vi "ZCR_enhanced_measurement_v6.vi"(8 "error in (no error)":errorcluster, 9 "Relay":enum16{"R1", "R2"}(ring), 10 "Serial Number":string, 11 "ZCR Signal Input":waveform(dbl)[](graph)=[{"t0"=timestamp(3707890383.8976955 s since 1904-01-01), "dt"=9.999999999999999e-05, "Y"=array[20000 elements], "attributes"=variant("NI_ChannelName"=variant(string "Tension_0"), "NI_UnitDescription"=variant(string "Volts"))}, {"t0"=timestamp(3707890383.8977456 s since 1904-01-01), "dt"=9.999999999999999e-05, "Y"=array[20000 elements], "attributes"=variant("NI_ChannelName"=variant(string "Tension_1"), "NI_UnitDescription"=variant(string "Volts"))}] caption="ZCR signal imput") -> (0 "error out":errorcluster, 1 "SIN OFF (x10)ms":dbl format="%0.2f", 2 "SIN ON (x10)ms":dbl format="%0.2f", 3 "ZCR measure OK ?":bool, 4 "Reglage decalage":T1={"Delta relais On (Secondes)"=0.002411111111111111, "Delta relais  Off(Secondes)"=0.0007555555555555556})   [LabVIEW 2020, in "Library Commun.lvlib" / "Nodon_ZCR.lvclass"]
uses:
  Nodon_ZCR.lvclass
  <vilib>/Utility/miscctls.llb/LVRangeTypeDef.ctl
  <vilib>/Analysis/baseanly.llb/Mean (DBL).vi
  <vilib>/Analysis/NI_AALBase.lvlib
  Library Commun.lvlib
panel:
  out "SIN ON Points":i32[](array[numeric])
  out "SIN OFF Points":i32[](array[numeric])
  out "ZCR OFF":waveform(dbl)[](graph)=[{"t0"=timestamp(3707890383.8976955 s since 1904-01-01), "dt"=9.999999999999999e-05, "Y"=array[20000 elements], "attributes"=variant("NI_ChannelName"=variant(string "Tension_0"), "NI_UnitDescription"=variant(string "Volts"))}, {"t0"=timestamp(3707890383.8977456 s since 1904-01-01), "dt"=9.999999999999999e-05, "Y"=array[20000 elements], "attributes"=variant("NI_ChannelName"=variant(string "Tension_1"), "NI_UnitDescription"=variant(string "Volts"))}]
  out "Input Signal":waveform(dbl)[](graph)=[{"t0"=timestamp(3810040522.776 s since 1904-01-01), "dt"=0.0002, "Y"=array[5000 elements]}, {"t0"=timestamp(3810040522.777 s since 1904-01-01), "dt"=0.0002, "Y"=array[5000 elements]}]
  out "SIN OFF Delay":i32[](array[numeric])
  out "SIN ON Delay":i32[](array[numeric])
  # "ZCR Enhanced V5"
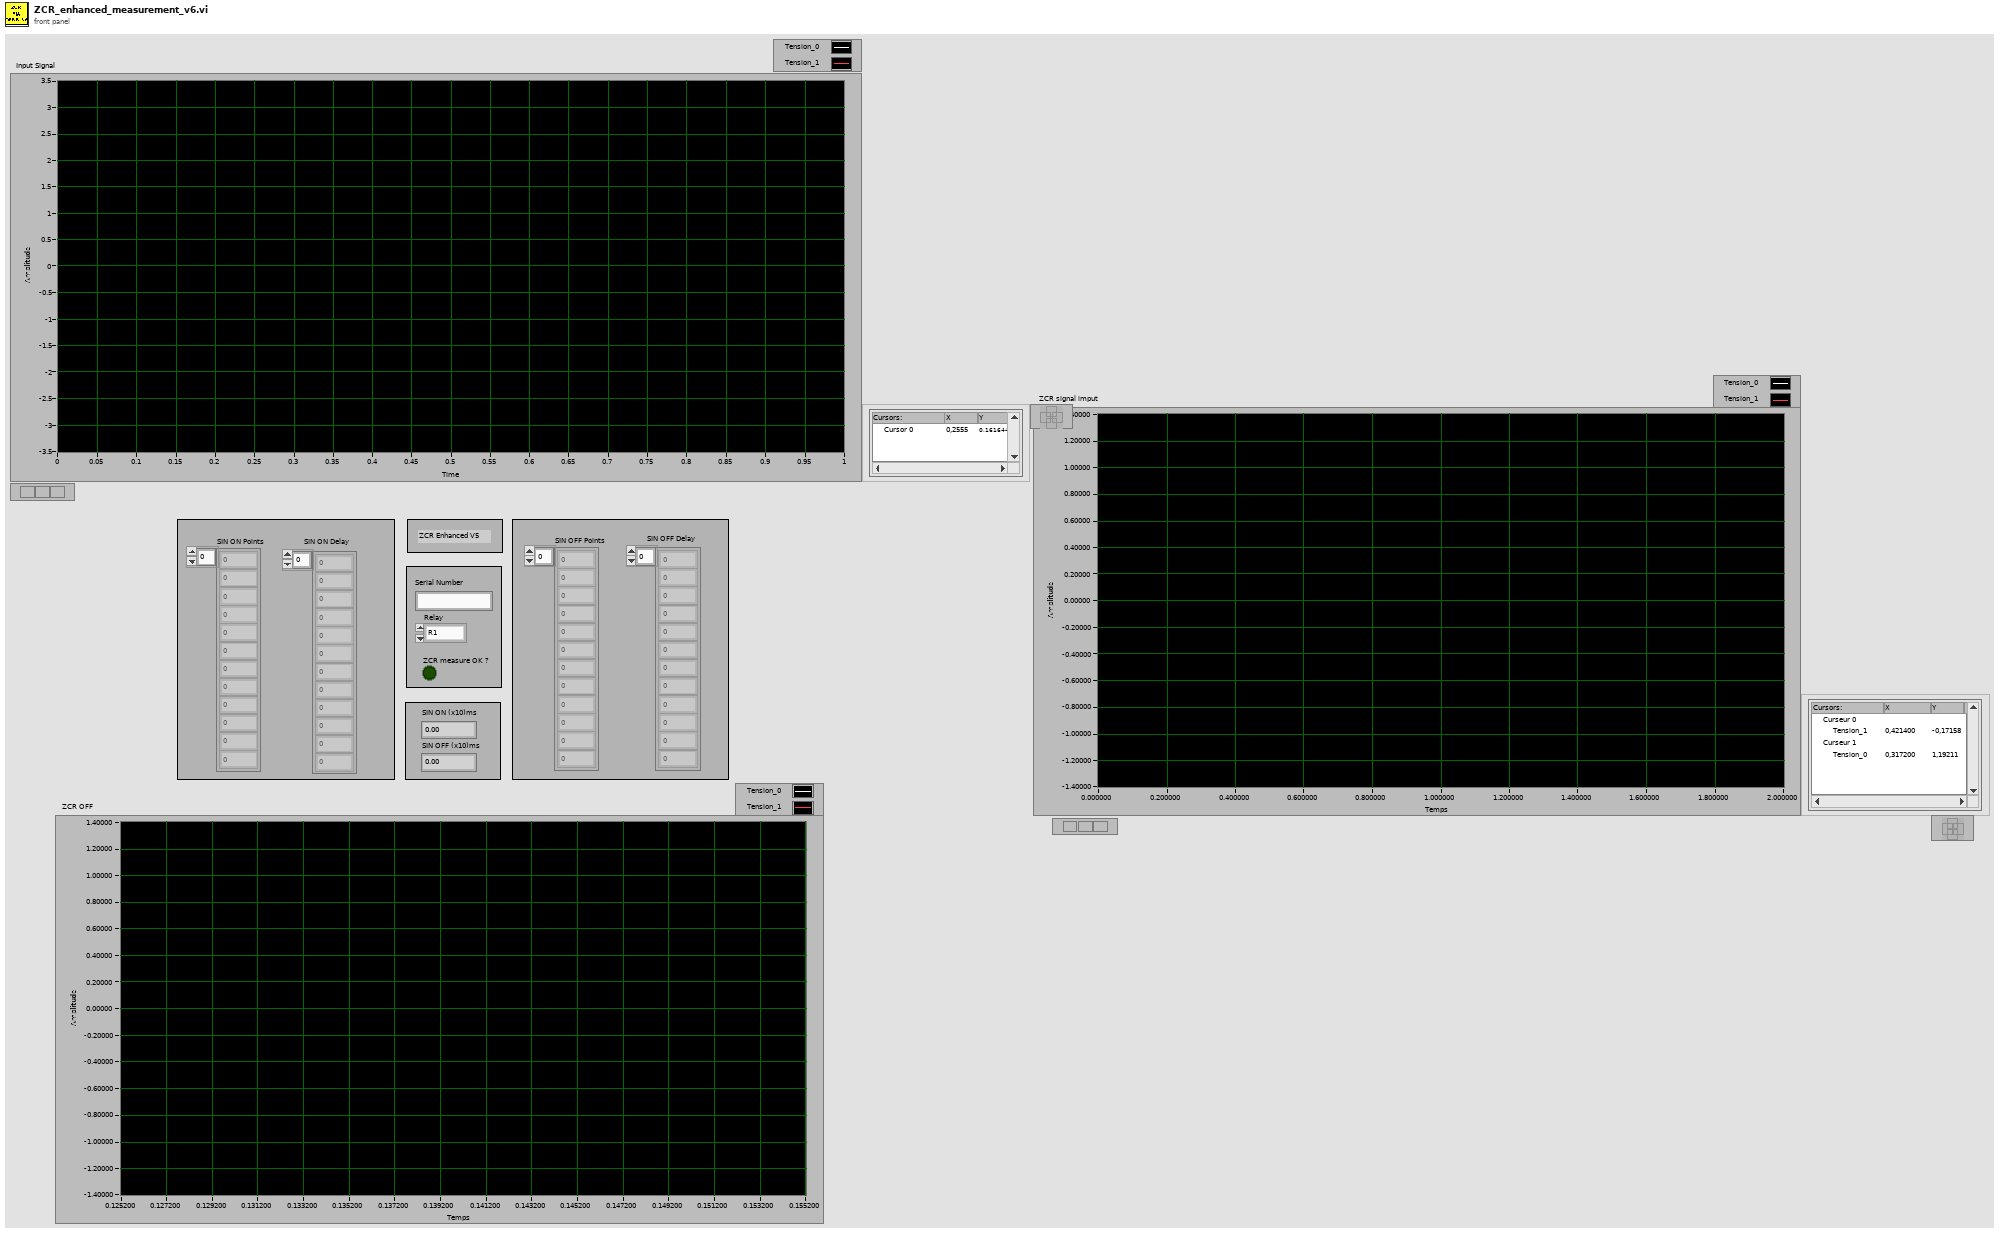
[diagram p1: front panel]
types:
  T1 = cluster{"Delta relais On (Secondes)":dbl, "Delta relais  Off(Secondes)":dbl}
  T2 = typedef "LVRangeTypeDef.ctl" = cluster{"Minimum":dbl, "Maximum":dbl, "Increment":dbl, "Minor Increment":dbl, "Start":dbl}
  T3 = typedef "imagedata.ctl" = cluster{"image type":i32, "image depth":i32, "image":u8[], "mask":u8[], "colors":u32[], "Rectangle":cluster{"left":i16, "top":i16, "right":i16, "bottom":i16}}
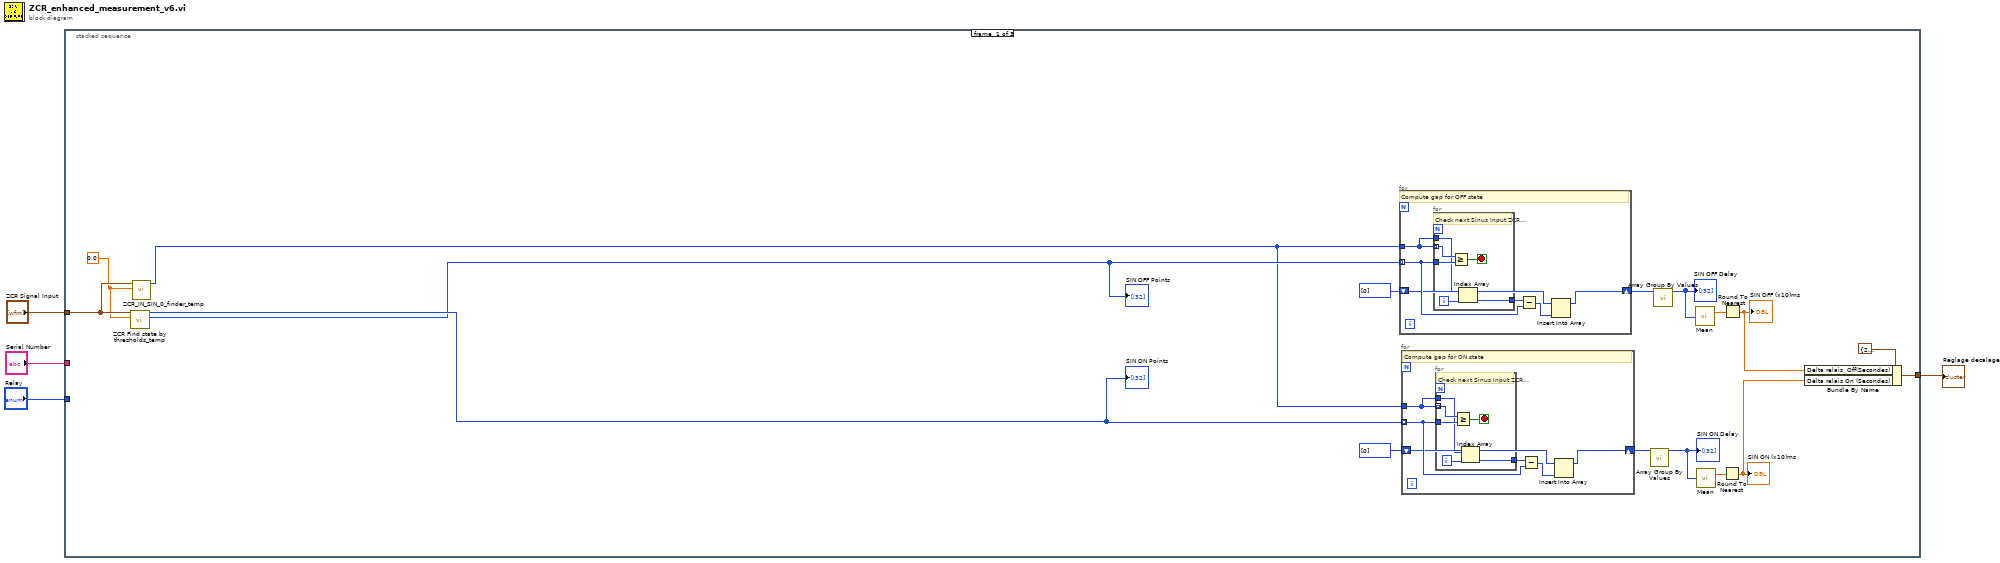
[diagram p0: block diagram]
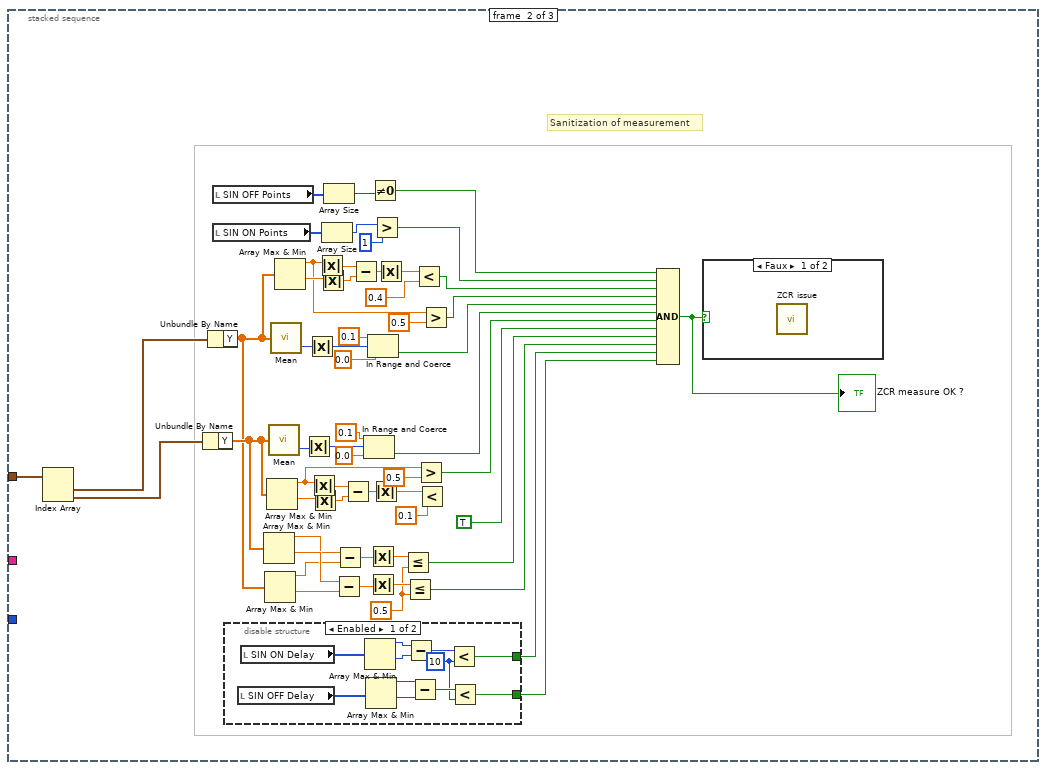
[diagram p2: hidden frame]
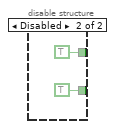
[diagram p3: hidden frame]
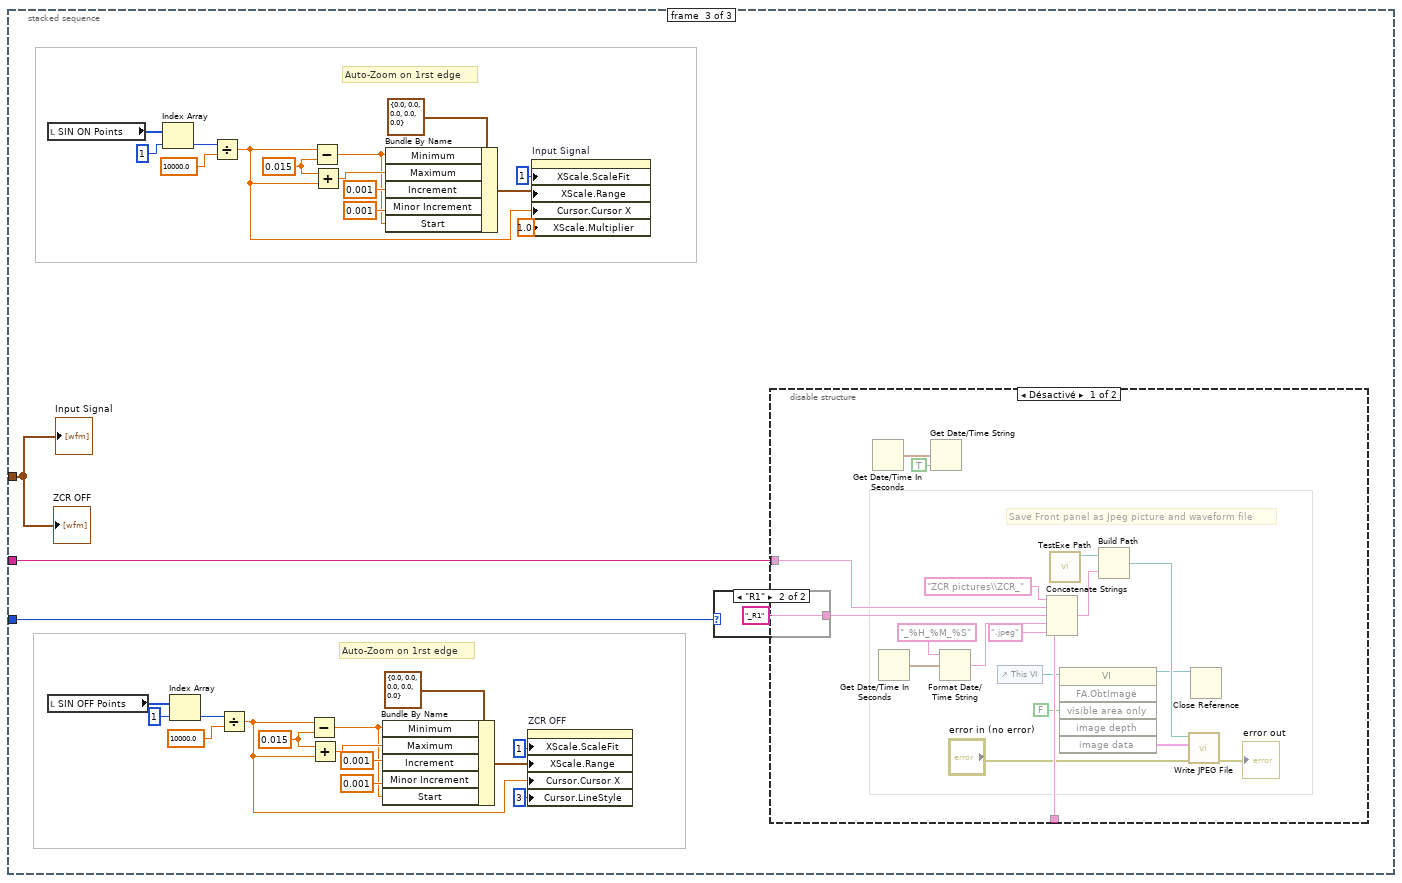
[diagram p5: hidden frame]
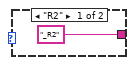
[diagram p7: hidden frame]
diagram:
  n1 = stacked-sequence {
    tunnel: "ZCR Signal Input" -> [w10 w47 w115]
    tunnel: "Serial Number" -> [_ _ w116]
    tunnel: "Relay" -> [_ _ w118]
    tunnel: [w15 _ _] -> w1
    frame #0 {
      w8 = 0.0
      n2 = call "ZCR Find state by thresholds_temp.vi"("Noise amplitude"=w8, "Input Signal"=w10) -> ("SIN OFF Points"=w11:i32[], "SIN ON Points"=w12:i32[])  [unwired: 8 in]
      "SIN OFF Points" <- w11
      "SIN ON Points" <- w12
      n3 = call "ZCR_IN_SIN_0_finder_temp.vi"("Noise amplitude"=w8, "ZCR IN"=w10) -> ("OFF SIN"=w9:i32[])  [unwired: 9 in]
      n4 = for {
        tunnel: w11 -> [w25] mode=indexing
        tunnel: w9 -> [w27]
        shift-right: [w22] -> w6
        shift-left: i32[] [0] -> [w24]
        # "Compute gap for OFF state"
        n5 = for {
          tunnel: w27 -> [w33] mode=indexing
          tunnel: w25 -> [w32]
          tunnel: w27 -> [w30]
          tunnel: [w29] -> w26
          i -> [w28]
          stop <- w31 stop-if-true
          # "Check next Sinus Input ZCR crossing"
          n6 = Greater Or Equal?(x=w33, y=w32) -> (x >= y?=w31:bool)
          n7 = Index Array(array=w30, index=w28) -> (element=w29:i32)
        }
        n8 = Subtract(x=w26, y=w25) -> (x-y=w23:i32)
        n9 = Insert Into Array(array=w24, new element=w23) -> (w22:i32[])  [unwired: 1 in]
      }
      n10 = for {
        tunnel: w12 -> [w37] mode=indexing
        tunnel: w9 -> [w39]
        shift-right: [w34] -> w19
        shift-left: i32[] [0] -> [w36]
        # "Compute gap for ON state"
        n11 = for {
          tunnel: w39 -> [w45] mode=indexing
          tunnel: w37 -> [w44]
          tunnel: w39 -> [w42]
          tunnel: [w41] -> w38
          i -> [w40]
          stop <- w43 stop-if-true
          # "Check next Sinus Input ZCR crossing"
          n12 = Greater Or Equal?(x=w45, y=w44) -> (x >= y?=w43:bool)
          n13 = Index Array(array=w42, index=w40) -> (element=w41:i32)
        }
        n14 = Subtract(x=w38, y=w37) -> (x-y=w35:i32)
        n15 = Insert Into Array(array=w36, new element=w35) -> (w34:i32[])  [unwired: 1 in]
      }
      n16 = call "Array Group By Values.vi"("Input Array"=w19) -> ("Output Value"=w7:i32[])  [unwired: 10 in]
      "SIN ON Delay" <- w7
      n17 = call "Array Group By Values.vi"("Input Array"=w6) -> ("Output Value"=w5:i32[])  [unwired: 10 in]
      "SIN OFF Delay" <- w5
      n18 = call-poly <vilib>:"Mean.vi"("X"=w5) -> ("mean"=w17:dbl)  [unwired: 1 out]
      n19 = call-poly <vilib>:"Mean.vi"("X"=w7) -> ("mean"=w18:dbl)  [unwired: 1 out]
      n20 = Round To Nearest(number=w18) -> (nearest integer value=w13:dbl)
      "SIN ON (x10)ms" <- w13
      n21 = Round To Nearest(number=w17) -> (nearest integer value=w14:dbl)
      "SIN OFF (x10)ms" <- w14
      n22 = Bundle By Name(cluster=T1 {"Delta relais On (Secondes)"=24.0, "Delta relais  Off(Secondes)"=7.0} ("Reglage decalage"), "Delta relais  Off(Secondes)"=w14, "Delta relais On (Secondes)"=w13) -> (w15:T1)
    }
    frame #1 {
      w55 = 0.5
      # "Sanitization of measurement"
      n23 = Index Array(array=w47) -> (element #1=w98:waveform(dbl), element #2=w97:waveform(dbl))  [unwired: 2 in]
      n24 = Unbundle By Name(w97) -> ("Y"=w65:dbl[])
      n25 = Unbundle By Name(w98) -> ("Y"=w64:dbl[])
      n26 = local read "SIN OFF Points"() -> (w101:i32[])
      n27 = local read "SIN ON Points"() -> (w100:i32[])
      n28 = disable-structure shown="Enabled" {
        disable-tunnel: [w103 TRUE] -> w49
        disable-tunnel: [w102 TRUE] -> w48
        frame Enabled {
          w104 = 10 ("y")
          n29 = local read "SIN OFF Delay"() -> (w111:i32[])
          n30 = local read "SIN ON Delay"() -> (w112:i32[])
          n31 = Array Max & Min(array=w112) -> (max value=w109:i32, min value=w110:i32)  [unwired: 2 out]
          n32 = Array Max & Min(array=w111) -> (max value=w107:i32, min value=w108:i32)  [unwired: 2 out]
          n33 = Subtract(x=w109, y=w110) -> (x-y=w106:i32)
          n34 = Subtract(x=w107, y=w108) -> (x-y=w105:i32)
          n35 = Less?(x=w106, y=w104) -> (x < y?=w103:bool)
          n36 = Less?(x=w105, y=w104) -> (x < y?=w102:bool)
        }
        frame Disabled {
        }
      }
      n37 = Array Max & Min(array=w65) -> (max value=w61:dbl, min value=w63:dbl)  [unwired: 2 out]
      n38 = Array Max & Min(array=w64) -> (max value=w60:dbl, min value=w62:dbl)  [unwired: 2 out]
      n39 = Array Max & Min(array=w65) -> (max value=w78:dbl, min value=w88:dbl)  [unwired: 2 out]
      n40 = call-poly <vilib>:"Mean.vi"("X"=w65) -> ("error"=w95:i32)  [unwired: 1 out]
      n41 = call-poly <vilib>:"Mean.vi"("X"=w64) -> ("error"=w96:i32)  [unwired: 1 out]
      n42 = Array Max & Min(array=w64) -> (max value=w75:dbl, min value=w83:dbl)  [unwired: 2 out]
      n43 = Absolute Value(x=w95) -> (abs(x)=w93:i32)
      n44 = Absolute Value(x=w96) -> (abs(x)=w94:i32)
      n45 = Absolute Value(x=w78) -> (abs(x)=w86:dbl)
      n46 = Absolute Value(x=w88) -> (abs(x)=w87:dbl)
      n47 = Absolute Value(x=w75) -> (abs(x)=w81:dbl)
      n48 = Absolute Value(x=w83) -> (abs(x)=w82:dbl)
      n49 = Array Size(array=w100) -> (size(s)=w51:i32)
      n50 = Array Size(array=w101) -> (size(s)=w99:i32)
      n51 = Subtract(x=w63, y=w62) -> (x-y=w58:dbl)
      n52 = Subtract(x=w61, y=w60) -> (x-y=w59:dbl)
      n53 = Subtract(x=w86, y=w87) -> (x-y=w85:dbl)
      n54 = Subtract(x=w81, y=w82) -> (x-y=w80:dbl)
      n55 = In Range and Coerce(upper limit=0.1, x=w93, lower limit=0.0) -> (In Range?=w69:bool)  [unwired: 1 out]
      n56 = In Range and Coerce(upper limit=0.1, x=w94, lower limit=0.0) -> (In Range?=w70:bool)  [unwired: 1 out]
      n57 = Absolute Value(x=w59) -> (abs(x)=w57:dbl)
      n58 = Absolute Value(x=w58) -> (abs(x)=w56:dbl)
      n59 = Not Equal To 0?(x=w99) -> (x != 0?=w74:bool)
      n60 = Absolute Value(x=w85) -> (abs(x)=w66:dbl)
      n61 = Greater?(x=w51, y=1) -> (0:w73:bool)
      n62 = Absolute Value(x=w80) -> (abs(x)=w67:dbl)
      n63 = Less Or Equal?(x=w57, y=w55) -> (x <= y?=w54:bool)
      n64 = Less Or Equal?(x=w56, y=w55) -> (x <= y?=w53:bool)
      n65 = Less?(x=w67, y=0.4) -> (x < y?=w72:bool)
      n66 = Greater?(x=w78, y=0.5) -> (0:w68:bool)
      n67 = Less?(x=w66, y=0.1) -> ()  [unwired: 1 out]
      n68 = Greater?(x=w75, y=0.5) -> (0:w71:bool)
      n69 = Compound Arithmetic op=AND(w74, w73, w72, w71, w70, w69, w68, TRUE, w54, w53, w49, w48) -> (w52:bool)
      "ZCR measure OK ?" <- w52
      n70 = case shown="Faux" w52 {
        frame False {
          n71 = call "ZCR issue"() -> ()  [unwired: 10 in, 2 out]
        }
        frame True {
        }
      }
    }
    frame #2 {
      w132 = 0.015
      w144 = 0.015
      # "Auto-Zoom on 1rst edge"
      # "Auto-Zoom on 1rst edge"
      n72 = local read "SIN ON Points"() -> (w138:i32[])
      n73 = local read "SIN OFF Points"() -> (w136:i32[])
      n74 = Index Array(array=w138, index=1) -> (element=w145:i32)
      n75 = Index Array(array=w136, index=1) -> (element=w133:i32)
      n76 = Divide(x=w145, y=10000.0) -> (x/y=w119:dbl)
      n77 = Divide(x=w133, y=10000.0) -> (x/y=w124:dbl)
      n78 = Subtract(x=w124, y=w132) -> (x-y=w127:dbl)
      n79 = Add(x=w132, y=w124) -> (x+y=w130:dbl)
      n80 = Subtract(x=w119, y=w144) -> (x-y=w139:dbl)
      n81 = Add(x=w144, y=w119) -> (x+y=w142:dbl)
      n82 = Bundle By Name(cluster=T2 {"Minimum"=0.0, "Maximum"=0.0, "Increment"=0.0, "Minor Increment"=0.0, "Start"=0.0} ("X Scale.Range"), "Minimum"=w127, "Maximum"=w130, "Increment"=0.001, "Minor Increment"=0.001, "Start"=w127) -> (w125:T2)
      n83 = Bundle By Name(cluster=T2 {"Minimum"=0.0, "Maximum"=0.0, "Increment"=0.0, "Minor Increment"=0.0, "Start"=0.0} ("X Scale.Range"), "Minimum"=w139, "Maximum"=w142, "Increment"=0.001, "Minor Increment"=0.001, "Start"=w139) -> (w122:T2)
      n84 = property on="ZCR OFF" class="GraphWF (strict)"("XScale.ScaleFit"=u8 1 ("X Scale.Scale Fit"), "XScale.Range"=w125, "Cursor.Cursor X"=w124, "Cursor.LineStyle"=u8 3 ("Cursor.Line Style")) -> ()  [unwired: 2 in, 2 out]
      n85 = property on="Input Signal" class="GraphWF (strict)"("XScale.ScaleFit"=u8 1 ("X Scale.Scale Fit"), "XScale.Range"=w122, "Cursor.Cursor X"=w119, "XScale.Multiplier"=1.0 ("X Scale.Offset and Multiplier:Multiplier")) -> ()  [unwired: 2 in, 2 out]
      n86 = case shown="\"R1\"" w118 {
        tunnel: ["_R2" "_R1"] -> w117
        frame "R2" {
        }
        frame "R1" {
        }
      }
      n87 = disable-structure shown="Désactivé" {
        disable-tunnel: w117 -> [w153 _]
        disable-tunnel: w116 -> [w152 _]
        frame Disabled {
          # "Save Front panel as Jpeg picture and waveform file"
          n88 = Get Date/Time In Seconds() -> (seconds since 1Jan1904=w151:timestamp)
          n89 = Get Date/Time In Seconds() -> (seconds since 1Jan1904=w156:timestamp)
          n90 = Get Date/Time String(seconds (now)=w151, want seconds? (F)=TRUE) -> ()  [unwired: 1 in, 2 out]
          n91 = Format Date/Time String(time format string (%c)="_%H_%M_%S", seconds (now)=w156) -> (date/time string=w154:string)  [unwired: 1 in]
          n92 = control-ref of="This VI"() -> (w161:refnum<vi>)
          n93 = Concatenate Strings("ZCR pictures\\ZCR_" ("nom ou chemin relatif"), w152, w153, w154, ".jpeg" ("nom ou chemin relatif")) -> (w148:string)
          n94 = call "TestExe Path.vi"() -> ("Chemin Actuel"=w147:path)  [unwired: 9 in, 2 out]
          n95 = invoke class="VI" method="FA.ObtImage"(reference=w161, "visible area only"=FALSE ("Visible Area Only")) -> (reference out=w159:refnum<vi>, "image data"=w162:T3)  [unwired: 4 in, 4 out]
          n96 = Build Path(base path=w147, name or relative path=w148) -> (appended path=w160:path)
          n97 = call <vilib>:"Write JPEG File.vi"("error in (no error)"="error in (no error)", "image data"=w162, "path to JPEG file"=w160) -> ("error out"=→"error out":errorcluster)  [unwired: 7 in, 1 out]
          n98 = Close Reference(reference=w159) -> ()  [unwired: 1 in, 1 out]
        }
        frame Enabled {
        }
      }
      "Input Signal" <- w115
      "ZCR OFF" <- w115
    }
  }
  "Reglage decalage" <- w1
